vi "SetAttribute.vi"(8 "error in (no error)":errorcluster, 10 "Set Attribute":T1, 11 "Data_Pupil_Diameter in":refnum<class "Data_Pupil.lvclass">) -> (0 "error out":errorcluster, 3 "Data_Pupil_Diameter out":refnum<class "Data_Pupil.lvclass">)   [LabVIEW 2020, in "Data_Pupil.lvclass"]
uses:
  Data_Pupil.lvclass
  Attribute.vi
  Data_Pupil.lvclass/Data_Pupil.ctl
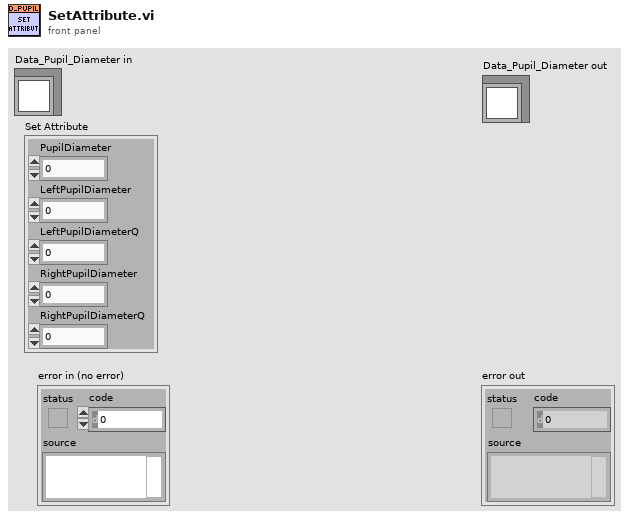
[diagram p1: front panel]
types:
  T1 = typedef "Data_Pupil.lvclass/Attribute.vi" = cluster{"PupilDiameter":dbl, "LeftPupilDiameter":dbl, "LeftPupilDiameterQ":dbl, "RightPupilDiameter":dbl, "RightPupilDiameterQ":dbl}
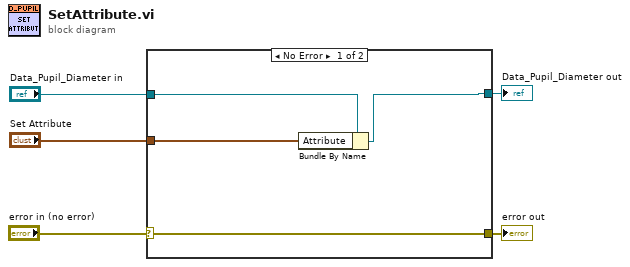
[diagram p0: block diagram]
diagram:
  n1 = case shown="No Error" "error in (no error)" {
    selector: "error in (no error)" -> [w9 w11]
    tunnel: [w9 w11] -> w4
    tunnel: [w7 w10] -> w3
    tunnel: "Data_Pupil_Diameter in" -> [w8 w10]
    tunnel: "Set Attribute" -> [w6 _]
    frame No Error {
      n2 = Bundle By Name(cluster=w8, "Attribute"=w6) -> (w7:refnum<class "Data_Pupil.lvclass">)
    }
    frame Error {
    }
  }
  "error out" <- w4
  "Data_Pupil_Diameter out" <- w3
